vi "PLC.File.Write.vi"(8 "error in":errorcluster, 11 "path":path) -> (0 "error out":errorcluster)   [LabVIEW 2016]
uses:
  Tools/Tma.lib/nlconfig.llb/fp2ini mode.ctl
  PLC.Global.vi
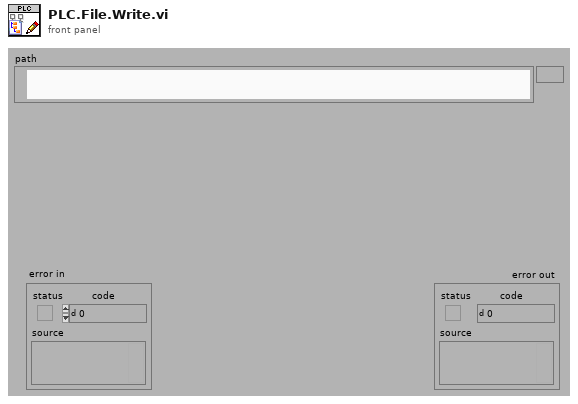
[diagram p1: front panel]
types:
  T1 = typedef "PLC.Data.Sets.ctl" = cluster{"Enable":bool, "IP":string, "Rack":i32, "Slot":i32, "LifeBitTimer_s":dbl, "DataBlockAddr_PCStatus":i32, "DataBlockAddr_PLCStatus":i32, "DataBlockAddr_PLCNewData":i32[], "DataBlockSize_PLCNewData":i32[], "DataBlockAddr_PLCChangeOver":i32[], "DataBlockSize_PLCChangeOver":i32[], "DataBlockAddr_PCChangeOver":i32[], "DataBlockAddr_PLCCheckStatus":i32[], "DataBlockSize_PLCCheckStatus":i32[], "DataBlockAddr_PCCheckStatus":i32[]}
  T2 = typedef "fp2ini mode.ctl" = enum16{"Read Controls", "Write Controls", "Write Indicators", "Read Indicators", "Write all", "Read all"}
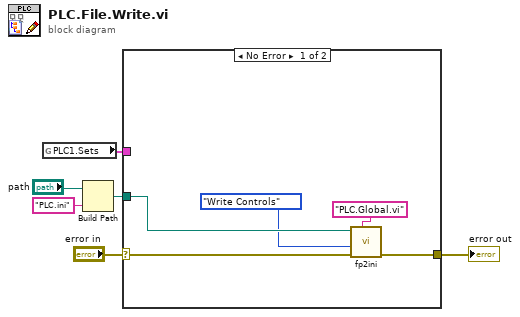
[diagram p0: block diagram]
diagram:
  n1 = global read "PLC.Global.vi" "PLC1.Sets"() -> (w1:T1)
  n2 = Build Path(base path="path", name or relative path="PLC.ini") -> (appended path=w3:path)
  n3 = case shown="No Error" "error in" {
    selector: "error in" -> [w11 w12]
    tunnel: [w8 w12] -> w6
    tunnel: w3 -> [w10 _]
    tunnel: w1 -> [_ _]
    frame No Error {
      n4 = call "fp2ini.vi"("vi-name (caller if empty)"="PLC.Global.vi", "error in"=w11, "mode"=fp2ini_mode."Write Controls", "ini-file path"=w10) -> ("error out"=w8:errorcluster)  [unwired: 3 in, 4 out]
    }
    frame Error {
    }
  }
  "error out" <- w6
